vi "Write Outgoing Bytes.vi"(8 "error in (no error)":errorcluster, 9 "timeout ms (2000)":i32=2000, 10 "Bytes":u8[](array[numeric]) format="%08b", 11 "LocalQueueConnection in":refnum<class "LocalQueueConnection.lvclass">) -> (0 "error out":errorcluster, 3 "LocalQueueConnection":refnum<class "LocalQueueConnection.lvclass">)   [LabVIEW 2013, in "MQTT_Queue.lvlib" / "LocalQueueConnection.lvclass"]
uses:
  LocalQueueConnection.lvclass
  LocalQueueConnection.lvclass/LocalQueueConnection.ctl
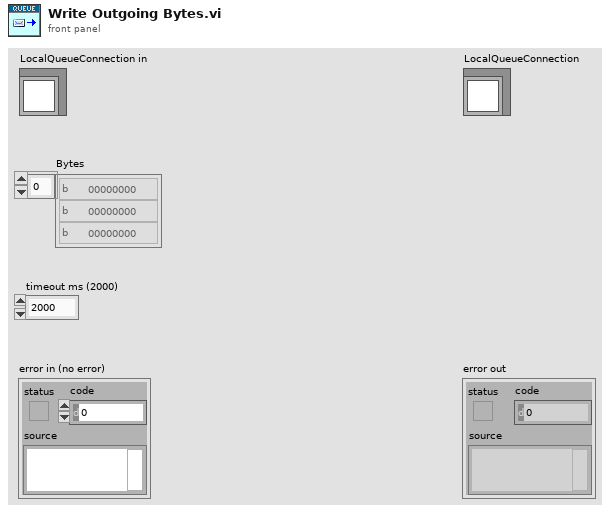
[diagram p1: front panel]
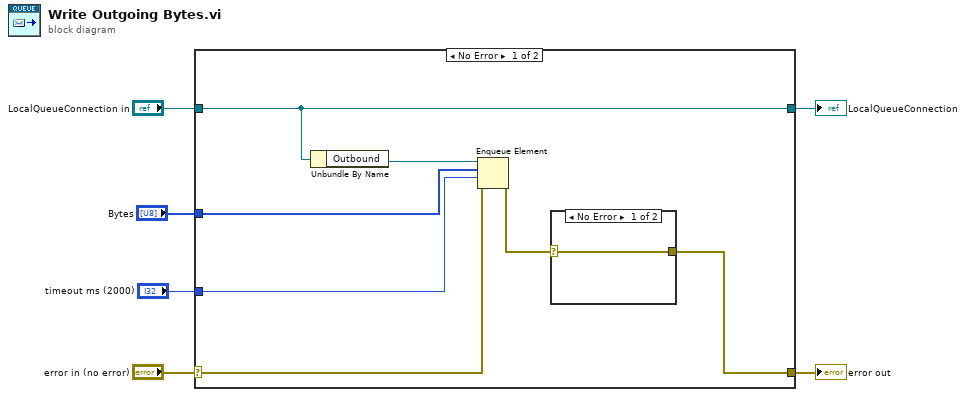
[diagram p0: block diagram]
diagram:
  n1 = case shown="No Error" "error in (no error)" {
    selector: "error in (no error)" -> [w9 w17]
    tunnel: [w12 w17] -> w5
    tunnel: [w13 w16] -> w3
    tunnel: "LocalQueueConnection in" -> [w13 w16]
    tunnel: "Bytes" -> [w10 _]
    tunnel: "timeout ms (2000)" -> [w7 _]
    frame No Error {
      n2 = Unbundle By Name(w13) -> ("Outbound"=w11:refnum<queue>)
      n3 = Enqueue Element(queue=w11, element=w10, timeout in ms (-1)=w7, error in (no error)=w9) -> (error out=w8:errorcluster)  [unwired: 2 out]
      n4 = case shown="No Error" w8 {
        selector: w8 -> [w14 w15]
        tunnel: [w14 w15] -> w12
        frame No Error {
        }
        frame Error {
        }
      }
    }
    frame Error {
    }
  }
  "error out" <- w5
  "LocalQueueConnection" <- w3
